vi "Save Keys.vi"(8 "error in (no error)":errorcluster, 11 "[MV] Key Generator in":refnum<class "[MV] Key Generator.lvclass">) -> (0 "error out":errorcluster, 3 "[MV] Key Generator out":refnum<class "[MV] Key Generator.lvclass">)   [LabVIEW 2020, in "[MV] Key Generator.lvlib" / "[MV] Key Generator.lvclass"]
uses:
  [MV] Key Generator.lvclass
  [MV] Key Generator.lvclass/[MV] Key Generator.ctl
  <vilib>/YU/Encrypt/AES/AES.lvclass
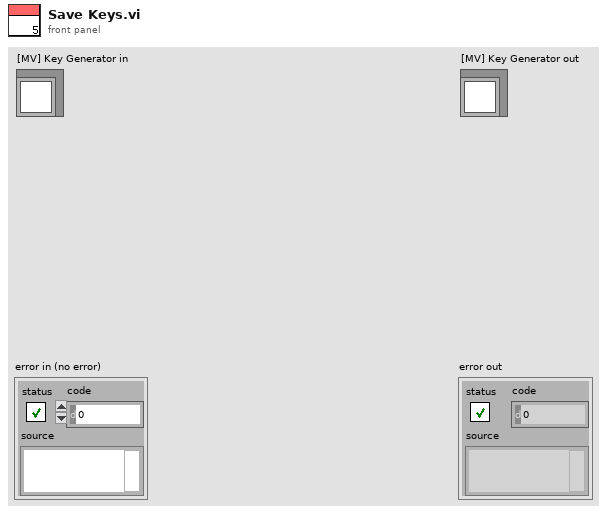
[diagram p1: front panel]
types:
  T1 = enum16{"open", "replace", "create", "open or create", "replace or create", "replace or create with confirmation"}
  T2 = map{string, cluster{"private":string, "public":string}}
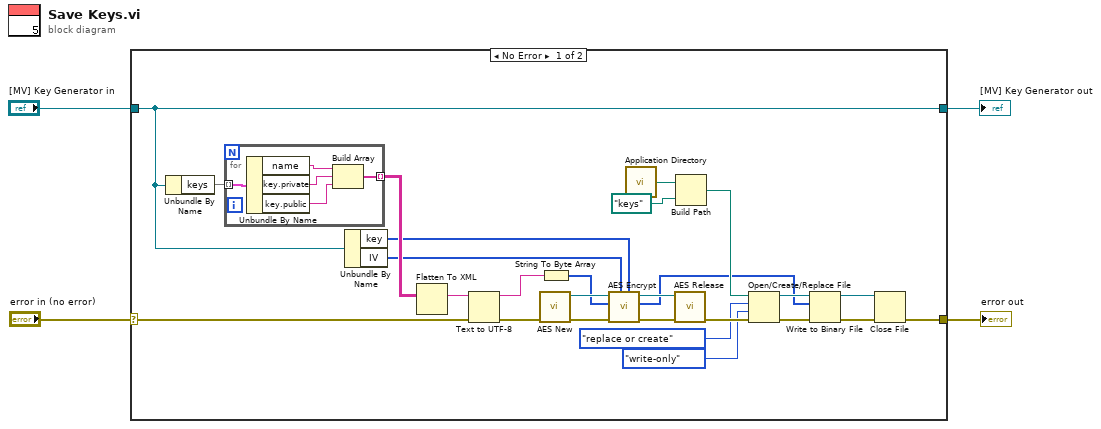
[diagram p0: block diagram]
diagram:
  n1 = case shown="No Error" "error in (no error)" {
    selector: "error in (no error)" -> [w5 w37]
    tunnel: [w6 w37] -> w3
    tunnel: [w24 w36] -> w1
    tunnel: "[MV] Key Generator in" -> [w24 w36]
    frame No Error {
      n2 = Unbundle By Name(w24) -> ("keys"=w30:T2)
      n3 = for {
        tunnel: w30 -> [w35] mode=indexing
        tunnel: [w31] -> w29 mode=indexing
        n4 = Unbundle By Name(w35) -> ("name"=w34:string, "key.private"=w33:string, "key.public"=w32:string)
        n5 = Build Array(w34, w33, w32) -> (w31:string[])
      }
      n6 = Unbundle By Name(w24) -> ("key"=w23:u8[], "IV"=w22:u8[])
      n7 = Flatten To XML(6:w29) -> (2:w28:string)
      n8 = Text to UTF-8(8:w5, 11:w28) -> (0:w27:errorcluster, 3:w21:string)  [unwired: 1 in]
      n9 = call <vilib>:"AES New.vi"("error in (no error)"=w27) -> ("error out"=w26:errorcluster, "AES out"=w25:refnum<class "AES.lvclass">)  [unwired: 9 in]
      n10 = String To Byte Array(string=w21) -> (unsigned byte array=w20:u8[])
      n11 = call <vilib>:"AES Encrypt.vi"("Key"=w23, "IV"=w22, "error in (no error)"=w26, "data"=w20, "AES in"=w25) -> ("error out"=w19:errorcluster, "encrypted data"=w9:u8[], "AES out"=w18:refnum<class "AES.lvclass">)  [unwired: 4 in]
      n12 = call <vilib>:"Application Directory.vi"() -> ("Application Directory"=w16:path)
      n13 = call <vilib>:"AES Release.vi"("error in (no error)"=w19, "AES in"=w18) -> ("error out"=w15:errorcluster)  [unwired: 9 in]
      n14 = Build Path(base path=w16, name or relative path=path "keys") -> (appended path=w14:path)
      n15 = Open/Create/Replace File(file path (use dialog)=w14, error in=w15, operation (0:open)=T1."replace or create", access (0:read/write)=enum16{"read/write", "read-only", "write-only"}."write-only") -> (refnum out=w10:refnum<file>, error out=w11:errorcluster)  [unwired: 2 in, 1 out]
      n16 = Write to Binary File(file (use dialog)=w10, data=w9, error in=w11) -> (refnum out=w7:refnum<file>, error out=w8:errorcluster)  [unwired: 3 in, 1 out]
      n17 = Close File(refnum=w7, error in=w8) -> (error out=w6:errorcluster)  [unwired: 1 out]
    }
    frame Error {
    }
  }
  "error out" <- w3
  "[MV] Key Generator out" <- w1
